vi "TCP-IP Link.Get Status.vi"(8 "error in":errorcluster, 11 "Link Q Name":string="TCP-IP_Link") -> (0 "error out":errorcluster)   [LabVIEW 2024, in "EQMF.lvlib" / "TCP-IP.lvlib"]
uses:
  TCP-IP.lvlib
  Queues/Queue Utils.lvlib
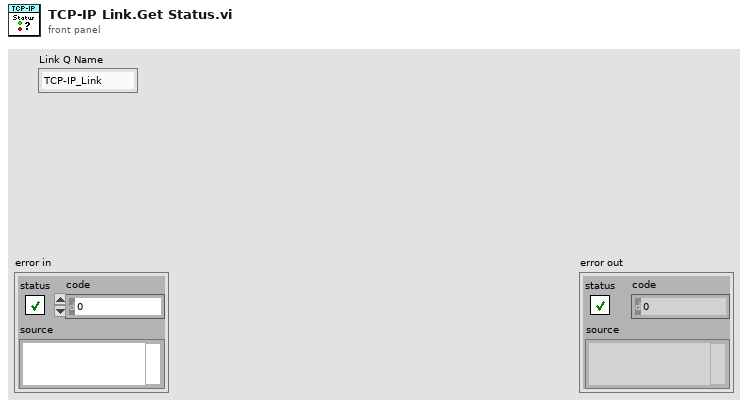
[diagram p1: front panel]
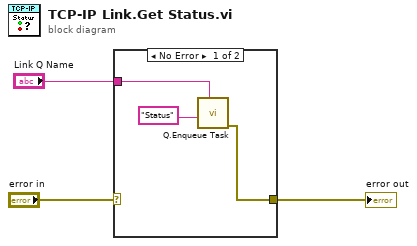
[diagram p0: block diagram]
diagram:
  n1 = case shown="No Error" "error in" {
    selector: "error in" -> [_ w7]
    tunnel: "Link Q Name" -> [w5 _]
    tunnel: [w4 w7] -> w1
    frame No Error {
      n2 = call "Q.Enqueue Task.vi"("Q Name"=w5, "Task Name"="Status") -> ("error out"=w4:errorcluster)  [unwired: 8 in, 1 out]
    }
    frame Error {
    }
  }
  "error out" <- w1
